vi "PathfinderUtil_ToTrajectory.vi"(11 "Pathfinder Path":T6[](array[typedef])) -> (3 "TRAJECTORY":T1 {"States"."POSE"."ROTATION"."SIN" format="%13.4f"; "States"."POSE"."ROTATION"."COS" format="%13.4f"; "States"."POSE"."ROTATION"."VALUE" format="%13.4f"; "States"."POSE"."TRANSLATION"."Y" format="%14.3f"; "States"."POSE"."TRANSLATION"."X" format="%14.3f"; "TotalTImeSecs" format="%20.3f"})   [LabVIEW 2019, in "Trajectory_Library.lvlib"]
doc: "This routine provides a complete conversion of a Pathfinder Path to a Trajectory. Each Pathfinder path sample is converted to a Trajectory State. The Trajectory states are optimied. (This is required to ensure that divide by zero doesn't occur when interpolating between states.) Then a Trajectory is created from the array of Trajectory states.\n\nParameters:\n - Pathfinder Path - Array of pathfinder created states\n\nReturns:\n - Trajectory - Trajectory data structure."
uses:
  Trajectory_Library.lvlib
  Pathfinder-Lib/VIs/Segment.ctl
  Pathfinder-Lib/Pathfinder.lvlib
  TypeDef/TRANSLATION2D.ctl
  TypeDef/ROTATION2D.ctl
  TypeDef/POSE2D.ctl
  TypeDef/TRAJ_STATE.ctl
  TypeDef/TRAJECTORY.ctl
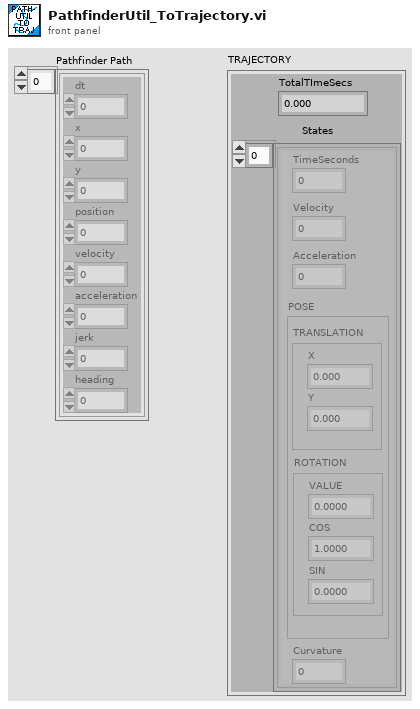
[diagram p1: front panel]
types:
  T1 = typedef "Trajectory_Library.lvlib/TRAJECTORY.ctl" = cluster{"TotalTImeSecs":dbl, "States":T2[]}
  T2 = typedef "Trajectory_Library.lvlib/TRAJ_STATE.ctl" = cluster{"TimeSeconds":dbl, "Velocity":dbl, "Acceleration":dbl, "POSE":T3, "Curvature":dbl}
  T3 = typedef "Trajectory_Library.lvlib/POSE2D.ctl" = cluster{"TRANSLATION":T4, "ROTATION":T5}
  T4 = typedef "Trajectory_Library.lvlib/TRANSLATION2D.ctl" = cluster{"X":dbl, "Y":dbl}
  T5 = typedef "Trajectory_Library.lvlib/ROTATION2D.ctl" = cluster{"VALUE":dbl, "COS":dbl, "SIN":dbl}
  T6 = typedef "Pathfinder.lvlib/Segment.ctl" = cluster{"dt":dbl, "x":dbl, "y":dbl, "position":dbl, "velocity":dbl, "acceleration":dbl, "jerk":dbl, "heading":dbl}
  T7 = typedef "WPILib_Math.lvlib/TRAJ_STATE.ctl" = cluster{"TimeSeconds":dbl, "Velocity":dbl, "Acceleration":dbl, "POSE":T8, "Curvature":dbl}
  T8 = typedef "WPILib_Math.lvlib/POSE2D.ctl" = cluster{"TRANSLATION":T9, "ROTATION":T10}
  T9 = typedef "WPILib_Math.lvlib/TRANSLATION2D.ctl" = cluster{"X":dbl, "Y":dbl}
  T10 = typedef "WPILib_Math.lvlib/ROTATION2D.ctl" = cluster{"VALUE":dbl, "COS":dbl, "SIN":dbl}
  T11 = typedef "WPILib_Math.lvlib/TRAJECTORY.ctl" = cluster{"TotalTImeSecs":dbl, "States":T7[]}
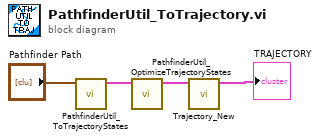
[diagram p0: block diagram]
diagram:
  n1 = call "PathfinderUtil_ToTrajectoryStates.vi"("Pathfinder Path"="Pathfinder Path") -> ("TrajectoryStates"=w4:T7[])  [unwired: 10 in]
  n2 = call "PathfinderUtil_OptimizeTrajectoryStates.vi"("inputTrajectoryStates"=w4) -> ("outputTrajectoryStates"=w2:T2[])  [unwired: 10 in]
  n3 = call "Trajectory_New.vi"("TRAJ_STATES"=w2) -> ("TRAJECTORY"=→"TRAJECTORY":T11)  [unwired: 10 in]
